vi "GPS Fix Quallity.vi"() -> ()   [LabVIEW 2016]
panel:
  in  "Fix Quality":i8
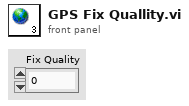
[diagram p1: front panel]
diagram:
